vi "writeToXML.vi"(8 "error in (no error)":errorcluster, 10 "ClassLabel":string, 11 "MccRotMove in":refnum<class "MccRotMove.lvclass">) -> (0 "error out":errorcluster, 2 "XMLout":string, 3 "MccRotMove out":refnum<class "MccRotMove.lvclass">)   [LabVIEW 2014, in "TCSDataDefinitions.lvlib" / "TCSMountControlCommand.lvlib" / "CommandsForRotatorAxis.lvlib" / "MccRotMove.lvclass"]
uses:
  MccRotMove.lvclass
  <userlib>/Common/UnitsAndXML/FlattenItemWithUnitToXML/FlattenPlaneAngleToXML/PlaneAngleUnit.ctl
  MccRotMove.lvclass/MccRotMove.ctl
  CommandsForRotatorAxis.lvclass
  <userlib>/Common/UnitsAndXML/UnitsAndXML.lvlib
  <userlib>/Common/XML/XMLGenerator/XMLGenerator.lvclass
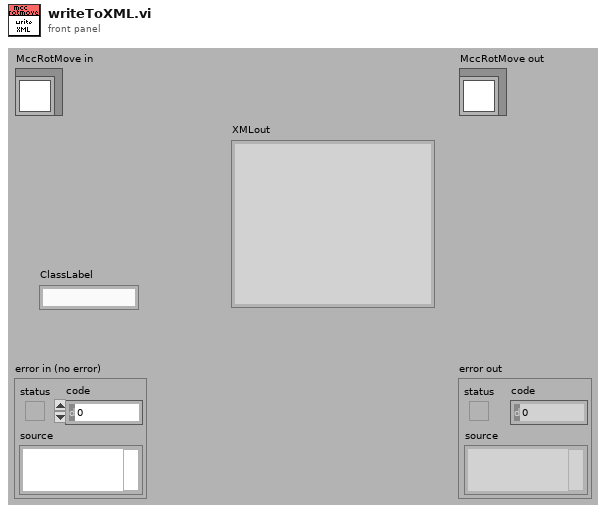
[diagram p1: front panel]
types:
  T1 = typedef "UnitsAndXML.lvlib/PlaneAngleUnit.ctl" = enum16{"rad", "deg", "'", "\""}
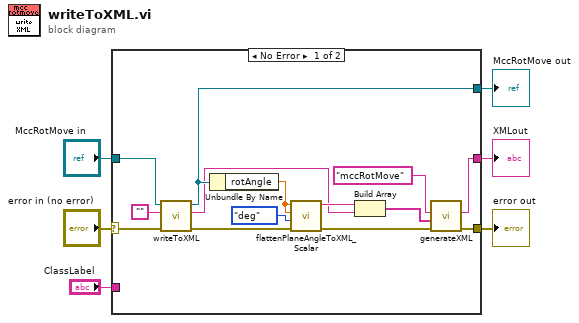
[diagram p0: block diagram]
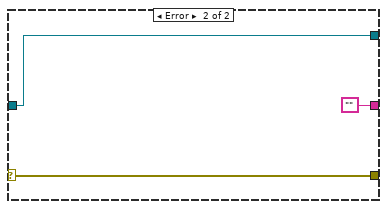
[diagram p2: hidden frame]
diagram:
  n1 = case shown="No Error" "error in (no error)" {
    selector: "error in (no error)" -> [w9 w23]
    tunnel: [w8 w23] -> w5
    tunnel: [w18 w22] -> w3
    tunnel: "MccRotMove in" -> [w19 w22]
    tunnel: "ClassLabel" -> [_ _]
    tunnel: [w7 ""] -> w1
    frame No Error {
      n2 = call-parent "writeToXML.vi"("error in (no error)"=w9, "ClassLabel"="", "CommandsForRotatorAxis in"=w19) -> ("error out"=w15:errorcluster, "XMLout"=w13:string, "CommandsForRotatorAxis out"=w18:refnum<class "MccRotMove.lvclass">)  [unwired: 6 in]
      n3 = Unbundle By Name(w18) -> ("rotAngle"=w17:dbl[unit])
      n4 = call <userlib>:"flattenPlaneAngleToXML_Scalar.vi"("error in (no error)"=w15, "planeAngleUnitInXML"=PlaneAngleUnit."deg", "planeAngleAgain"=w17, "planeAngle"=w17) -> ("error out"=w10:errorcluster, "xmlString"=w14:string)  [unwired: 6 in]
      n5 = Build Array(w14, w13) -> (w12:string[])
      n6 = call <userlib>:"generateXML.vi"("error in"=w10, "childrenXML"=w12, "elementName"="mccRotMove" ("Class Label")) -> ("error out"=w8:errorcluster, "XML out"=w7:string)  [unwired: 6 in, 1 out]
    }
    frame Error {
    }
  }
  "error out" <- w5
  "MccRotMove out" <- w3
  "XMLout" <- w1
